vi "Main.vi"(8 "error in":errorcluster, 11 "ModuleA in":refnum<class "ModuleA.lvclass">) -> (0 "error out":errorcluster, 3 "ModuleA out":refnum<class "ModuleA.lvclass">)   [LabVIEW 2019, in "ModuleA.lvclass"]
doc: "The <b>Queued Message Handler</b> of the Worker that owns this VI."
uses:
  ModuleA.lvclass
  ModuleA.lvclass/ModuleA.ctl
  Initialization Data.ctl
  Response Cases.ctl
  rwr_RequestMeasureData.ctl
  <vilib>/addons/_Workers/Library/Case Label.ctl
  <vilib>/addons/_Workers/Library/Workers.lvlib
  rql_ReadMeasureDataProcess.ctl
  <vilib>/measure/NI_MABase.lvlib
  dab2204b-7db6-4626-b970-28036f5fd160.vi
  rwr_RequestMeasureData Reply.ctl
panel:
  out "Waveform Graph":waveform(dbl)(graph)
  out "Progress":u8(slide) scale=0.0..100.0
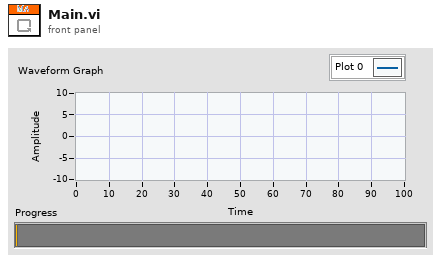
[diagram p1: front panel]
types:
  T1 = typedef "ModuleA.lvclass/Initialization Data.ctl" = cluster{"Response Cases":T2}
  T2 = typedef "ModuleA.lvclass/Response Cases.ctl" = cluster{"Placeholder - Can be deleted":string, "FeedbackMA_Data":T3}
  T3 = typedef "Workers.lvlib/Case Label.ctl" = string
  T4 = typedef "ModuleA.lvclass/rql_ReadMeasureDataProcess.ctl" = cluster{"String":string}
  T5 = typedef "ModuleA.lvclass/rwr_RequestMeasureData Reply.ctl" = cluster{"String":string, "Waveform":waveform(dbl)}
  T6 = typedef "ModuleA.lvclass/rwr_RequestMeasureData.ctl" = cluster{"String":string}
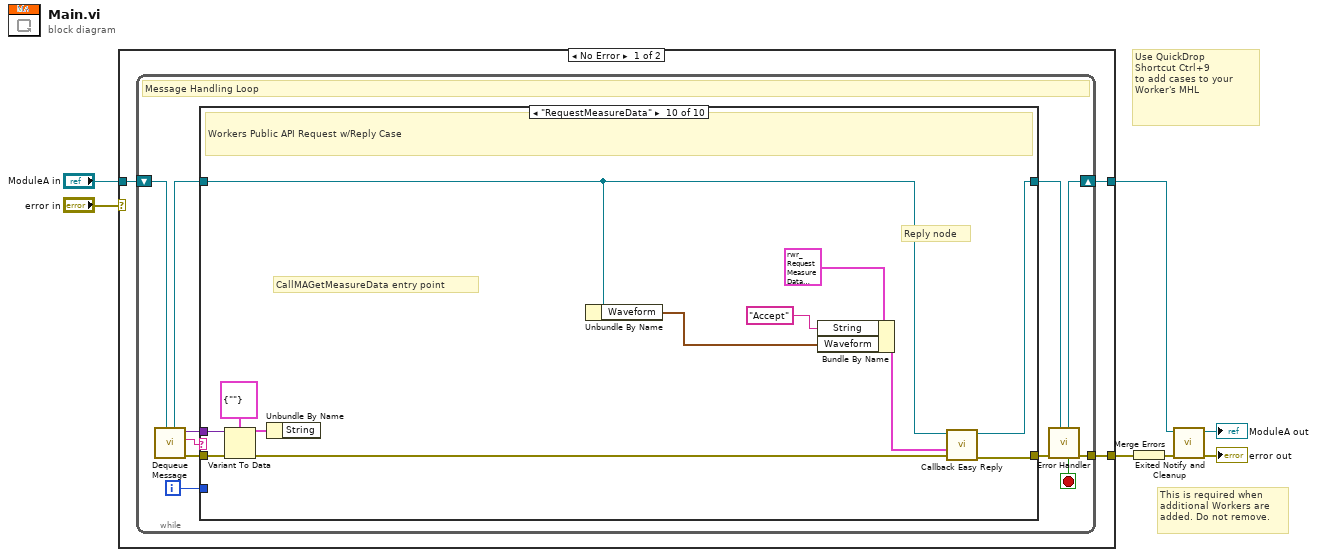
[diagram p0: block diagram]
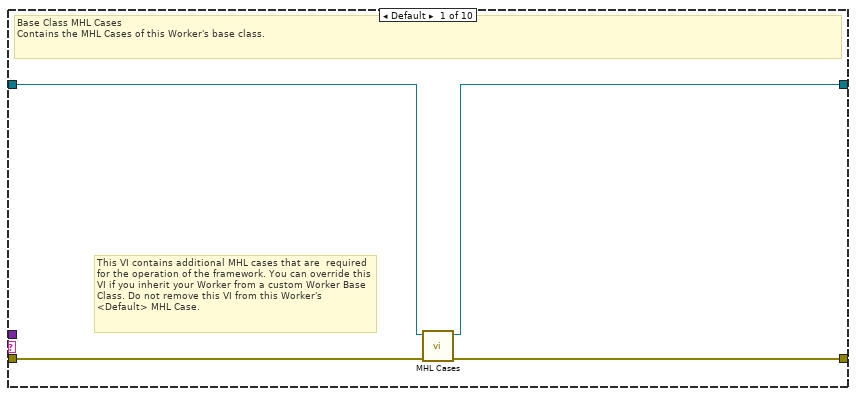
[diagram p2: hidden frame]
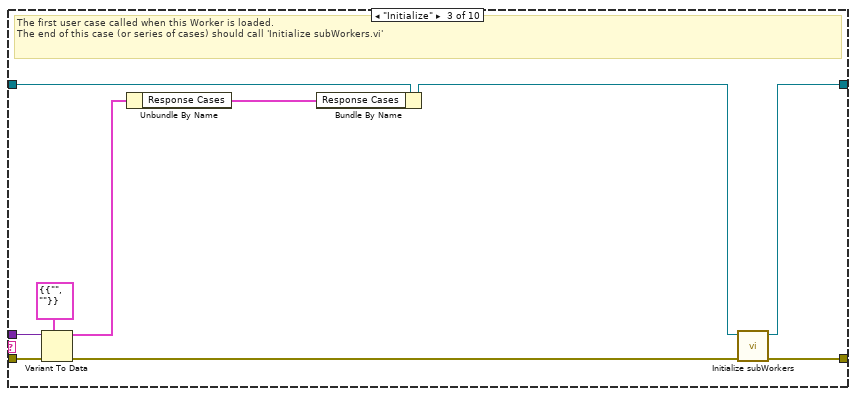
[diagram p4: hidden frame]
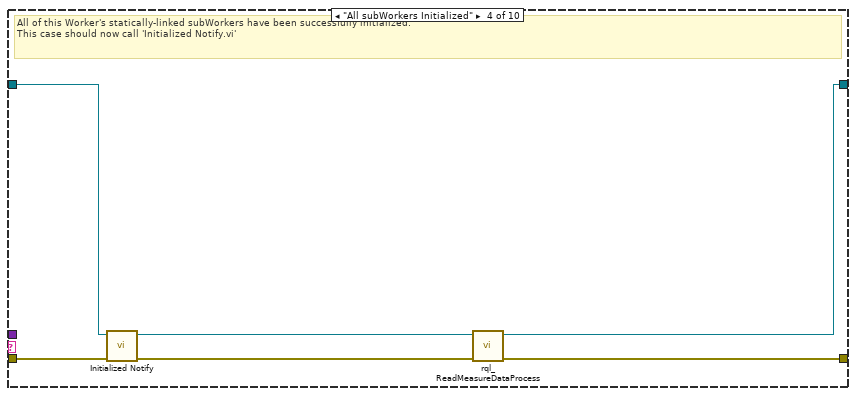
[diagram p5: hidden frame]
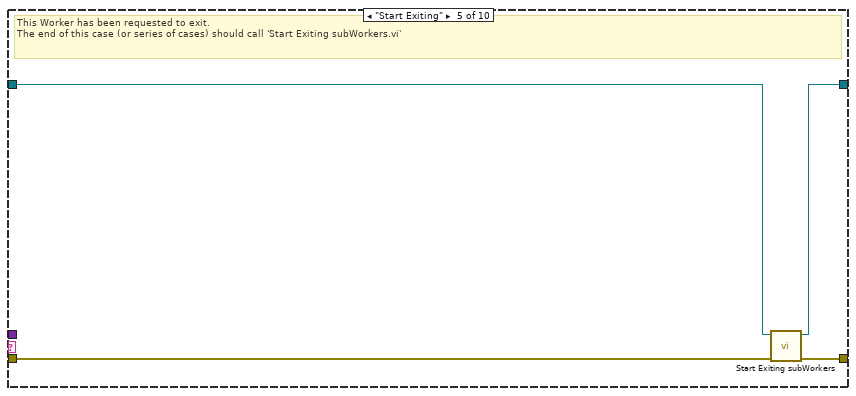
[diagram p6: hidden frame]
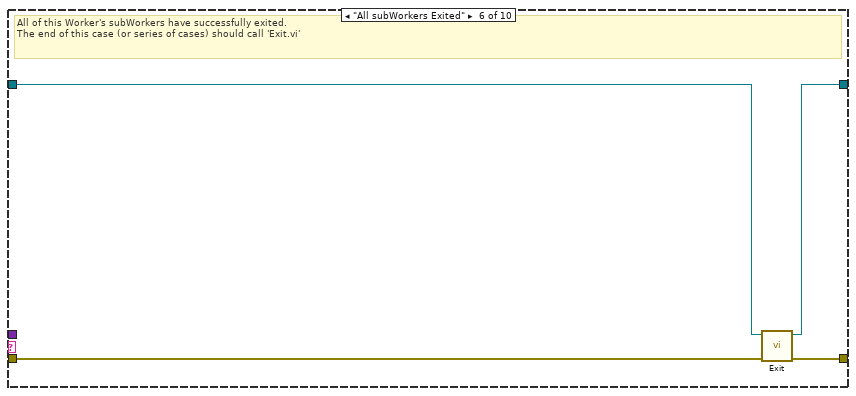
[diagram p7: hidden frame]
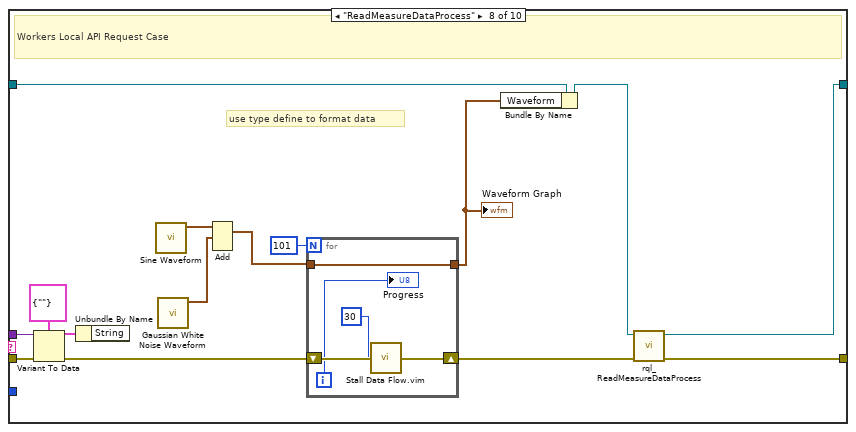
[diagram p9: hidden frame]
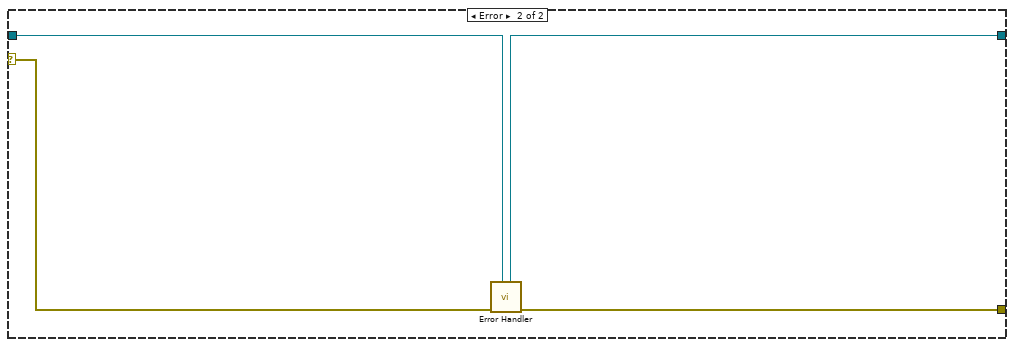
[diagram p11: hidden frame]
diagram:
  # "Use QuickDrop\nShortcut Ctrl+9\nto add cases to your\nWorker's MHL"
  # "This is required when additional Workers are added. Do not remove."
  n1 = case shown="No Error" "error in" {
    tunnel: "ModuleA in" -> [w8 w89]
    tunnel: [w10 w90] -> w6
    tunnel: [w9 w88] -> w7
    selector: "error in" -> [_ w91]
    frame No Error {
      n2 = while {
        shift-right: [w19] -> w9
        shift-left: w8 -> [w21]
        tunnel: [w20] -> w10
        i -> [w12]
        stop <- w13 stop-if-true
        # "Message Handling Loop"
        n3 = call-dynamic "Dequeue Message.vi"("Worker"=w21) -> ("error out"=w18:errorcluster, "Case out"=w14:string, "Data out"=w11:variant, "Worker out"=w16:refnum<class "ModuleA.lvclass">)  [unwired: 6 in, 1 out]
        n4 = case "Worker MHL Case Structure (DO NOT CHANGE LABEL NAME)" shown="\"RequestMeasureData\"" w14 {
          tunnel: w18 -> [w25 w26 w35 w43 w44 w51 w53 w68 w75 w87]
          tunnel: [w24 w26 w37 w40 w47 w50 w53 w58 w75 w78] -> w17
          tunnel: w16 -> [w23 w27 w34 w41 w45 w49 w52 w57 w74 w77]
          tunnel: [w22 w27 w36 w38 w46 w48 w52 w56 w74 w79] -> w15
          tunnel: w12 -> [_ _ _ _ _ _ _ _ _ _]
          tunnel: w11 -> [_ _ w32 _ _ _ _ w65 _ w84]
          frame Default {
            # "This VI contains additional MHL cases that are  required for the operation of the framework. You can override this VI if you inherit your Worker from a custom Worker Base Class. Do not remove this VI from this Worker's <Default> MHL Case."
            # "Base Class MHL Cases\nContains the MHL Cases of this Worker's base class."
            n5 = call-dynamic "MHL Cases.vi"("error in"=w25, "Worker in"=w23) -> ("error out"=w24:errorcluster, "Worker out"=w22:refnum<class "ModuleA.lvclass">)  [unwired: 8 in]
          }
          frame "------------ FRAMEWORK CASES -----------" {
            # "Start of Workers Framework Cases"
          }
          frame "Initialize" {
            # "The first user case called when this Worker is loaded.\nThe end of this case (or series of cases) should call 'Initialize subWorkers.vi'"
            n6 = Variant To Data(error in=w35, type=T1 {"Response Cases"={"Placeholder - Can be deleted"="", "FeedbackMA_Data"=""}} ("Cluster"), Variant=w32) -> (data=w30:T1, error out=w33:errorcluster)
            n7 = Unbundle By Name(w30) -> ("Response Cases"=w29:T2)
            n8 = Bundle By Name(cluster=w34, "Response Cases"=w29) -> (w31:refnum<class "ModuleA.lvclass">)
            n9 = call-dynamic "Initialize subWorkers.vi"("error in"=w33, "Worker"=w31) -> ("error out"=w37:errorcluster, "dup Worker out"=w36:refnum<class "ModuleA.lvclass">)  [unwired: 8 in]
          }
          frame "All subWorkers Initialized" {
            # "All of this Worker's statically-linked subWorkers have been successfully initialized.\nThis case should now call 'Initialized Notify.vi'"
            n10 = call-dynamic "Initialized Notify.vi"("error in"=w43, "Worker"=w41) -> ("error out"=w42:errorcluster, "dup Worker out"=w39:refnum<class "ModuleA.lvclass">)  [unwired: 8 in]
            n11 = call "rql_ReadMeasureDataProcess.vi"("error in"=w42, "ModuleA in"=w39) -> ("error out"=w40:errorcluster, "dup ModuleA out"=w38:refnum<class "ModuleA.lvclass">)  [unwired: 8 in]
          }
          frame "Start Exiting" {
            # "This Worker has been requested to exit. \nThe end of this case (or series of cases) should call 'Start Exiting subWorkers.vi'"
            n12 = call-dynamic "Start Exiting subWorkers.vi"("error_in"=w44, "Worker"=w45) -> ("error out"=w47:errorcluster, "dup Worker out"=w46:refnum<class "ModuleA.lvclass">)  [unwired: 8 in]
          }
          frame "All subWorkers Exited" {
            # "All of this Worker's subWorkers have successfully exited. \nThe end of this case (or series of cases) should call 'Exit.vi'"
            n13 = call-dynamic "Exit.vi"("error_in"=w51, "Worker"=w49) -> ("error out"=w50:errorcluster, "dup Worker out"=w48:refnum<class "ModuleA.lvclass">)  [unwired: 8 in]
          }
          frame "------------- LOCAL API CASES -------------" {
            # "Start of Workers Local API Cases"
          }
          frame "ReadMeasureDataProcess" {
            # "use type define to format data"
            # "Workers Local API Request Case"
            n14 = Variant To Data(error in=w68, type=T4 {"String"=""} ("Data"), Variant=w65) -> (data=w64:T4, error out=w67:errorcluster)
            n15 = Unbundle By Name(w64) -> ()  [unwired: 1 out]
            n16 = call <vilib>:"Sine Waveform.vi"() -> ("signal out"=w63:waveform(dbl))  [unwired: 10 in, 1 out]
            n17 = call <vilib>:"Gaussian White Noise Waveform.vi"() -> ("signal out"=w62:waveform(dbl))  [unwired: 10 in, 1 out]
            n18 = Add(1:w62, 2:w63) -> (0:w59:waveform(dbl))  [unwired: 1 in, 1 out]
            n19 = for {
              N: 101 -> [_]
              shift-right: [w72] -> w61
              shift-left: w67 -> [w73]
              tunnel: [w69] -> w54
              tunnel: w59 -> [w69]
              i -> [w70]
              n20 = call "Stall Data Flow.vim"("value in"=w73, "milliseconds to wait"=u32 30) -> ("value out"=w72:errorcluster)  [unwired: 1 out]
              "Progress" <- w70
            }
            "Waveform Graph" <- w54
            n21 = Bundle By Name(cluster=w57, "Waveform"=w54) -> (w55:refnum<class "ModuleA.lvclass">)
            n22 = call "rql_ReadMeasureDataProcess.vi"("error in"=w61, "ModuleA in"=w55) -> ("error out"=w58:errorcluster, "dup ModuleA out"=w56:refnum<class "ModuleA.lvclass">)  [unwired: 8 in]
          }
          frame "------------- PUBLIC API CASES -------------" {
            # "Start of Workers Public API Cases"
          }
          frame "RequestMeasureData" {
            # "Reply node"
            # "CallMAGetMeasureData entry point"
            # "Workers Public API Request w/Reply Case"
            n23 = Variant To Data(error in=w87, type=T6 {"String"=""} ("Data"), Variant=w84) -> (data=w83:T6, error out=w86:errorcluster)
            n24 = Unbundle By Name(w83) -> ()  [unwired: 1 out]
            n25 = Unbundle By Name(w77) -> ("Waveform"=w76:waveform(dbl))
            n26 = Bundle By Name(cluster=T5 {"String"="", "Waveform"={"t0"=timestamp(0 s since 1904-01-01), "dt"=1.0, "Y"=[]}} ("Reply Data"), "String"="Accept", "Waveform"=w76) -> (w81:T5)
            n27 = call-dynamic "Callback Easy Reply.vi"("error in"=w86, "Data"=w81, "Worker"=w77) -> ("error out"=w78:errorcluster, "dup Worker out"=w79:refnum<class "ModuleA.lvclass">)  [unwired: 7 in]
          }
        }
        n28 = call-dynamic "Error Handler.vi"("Worker"=w15, "error_in"=w17) -> ("error out"=w20:errorcluster, "Stop Loop"=w13:bool, "Worker out"=w19:refnum<class "ModuleA.lvclass">)  [unwired: 7 in]
      }
    }
    frame Error {
      n29 = call-dynamic "Error Handler.vi"("Worker"=w89, "error_in"=w91) -> ("error out"=w90:errorcluster, "Worker out"=w88:refnum<class "ModuleA.lvclass">)  [unwired: 7 in, 1 out]
    }
  }
  n30 = Merge Errors(w6) -> (w3:errorcluster)
  n31 = call-dynamic "Exited Notify and Cleanup.vi"("error_in"=w3, "Worker"=w7) -> ("error out"=→"error out":errorcluster, "dup Worker out"=→"ModuleA out":refnum<class "ModuleA.lvclass">)  [unwired: 8 in]
